vi "Draw Tree.vi"(8 "error in (no error)":errorcluster, 10 "Tree Data":T1(array[cluster]), 11 "Test Executive Builder View in":refnum<class "Test Executive Builder View.lvclass">) -> (0 "error out":errorcluster, 3 "Test Executive Builder View out":refnum<class "Test Executive Builder View.lvclass">)   [LabVIEW 2017, in "Test Executive Builder View.lvclass"]
uses:
  <vilib>/gpm_packages/@cs/Test-executive-builder/Source/Test Executive Builder View/Test Executive Builder View/Test Executive Builder View.lvclass
  <vilib>/gpm_packages/@cs/Test-executive-builder/Source/Test Executive Builder View/Test Executive Builder View/Test Executive Builder View.lvclass/Test Executive Builder View.ctl
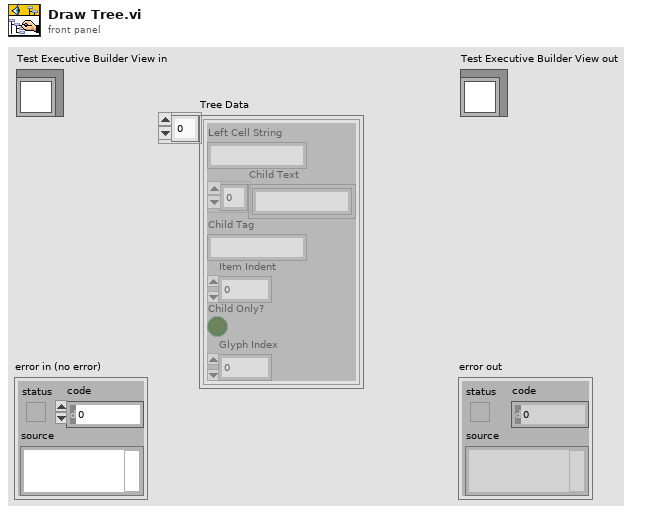
[diagram p1: front panel]
types:
  T1 = cluster{"Left Cell String":string, "Child Text":string[], "Child Tag":string, "Item Indent":i32, "Child Only?":bool, "Glyph Index":i32}[]
  T2 = typedef "LVNodeAndColumnTypeDef.ctl" = cluster{"Node":string, "Column":i32}
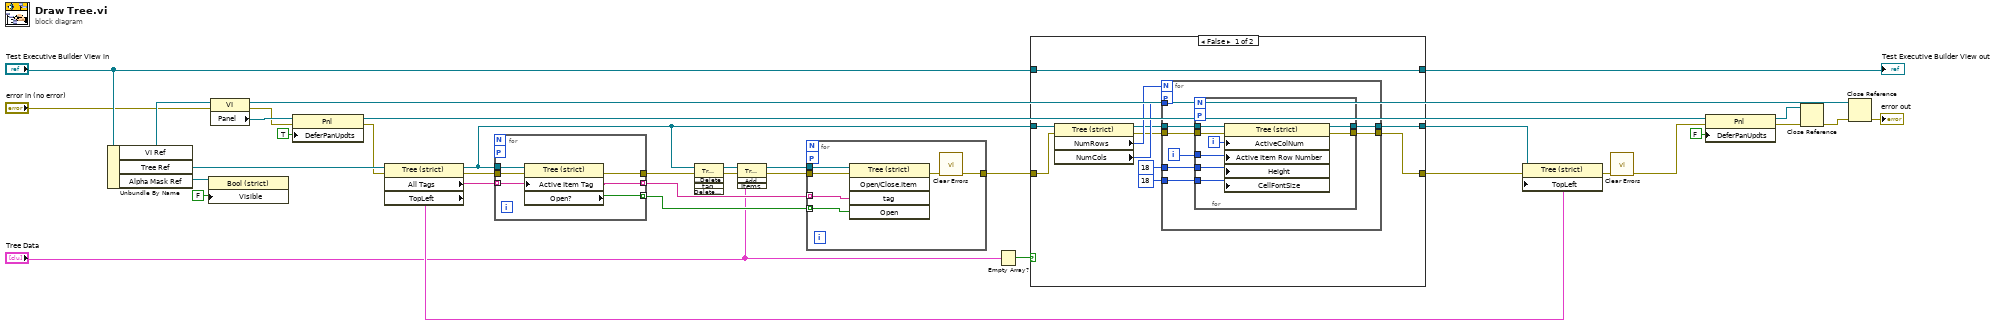
[diagram p0: block diagram]
diagram:
  n1 = Unbundle By Name("Test Executive Builder View in") -> ("VI Ref"=w36:refnum<vi>, "Tree Ref"=w32:refnum<vi>, "Alpha Mask Ref"=w11:refnum<vi>)
  n2 = property class="Bool (strict)"(reference=w11, "Visible"=FALSE) -> ()  [unwired: 1 in, 2 out]
  n3 = property class="VI"(reference=w36, error in="error in (no error)") -> (reference out=w15:refnum<vi>, error out=w33:errorcluster, "Panel"=w35:refnum<vi>)
  n4 = property class="Pnl"(reference=w35, error in=w33, "DeferPanUpdts"=TRUE ("Defer Panel Updates")) -> (reference out=w18:refnum<vi>, error out=w31:errorcluster)
  n5 = property class="Tree (strict)"(reference=w32, error in=w31) -> (reference out=w2:refnum<vi>, error out=w30:errorcluster, "All Tags"=w29:string[], "TopLeft"=w8:T2)
  n6 = for {
    tunnel: w29 -> [w37] mode=indexing
    tunnel: [w38] -> w23 mode=indexing
    tunnel: [w37] -> w22 mode=indexing
    tunnel: w30 -> [w40]
    tunnel: [w39] -> w28
    tunnel: w2 -> [w41]
    workers-P: _ -> [_]
    n7 = property class="Tree (strict)"(reference=w41, error in=w40, "Active Item Tag"=w37) -> (error out=w39:errorcluster, "Open?"=w38:bool)  [unwired: 1 out]
  }
  n8 = invoke class="Tree (strict)" method="Edit Tree Items.Delete"(reference=w2, error in=w28) -> (reference out=w27:refnum<vi>, error out=w26:errorcluster)  [unwired: 3 in, 3 out]
  n9 = invoke class="Tree (strict)" method="Edit Tree Items.Add Multiple Items to End"(reference=w27, error in=w26, "Items"="Tree Data") -> (reference out=w24:refnum<vi>, error out=w25:errorcluster)  [unwired: 1 in, 2 out]
  n10 = for {
    tunnel: w24 -> [w46]
    tunnel: w22 -> [w44] mode=indexing
    tunnel: w23 -> [w43] mode=indexing
    tunnel: w25 -> [w47]
    tunnel: [w42] -> w3
    workers-P: _ -> [_]
    n11 = invoke class="Tree (strict)" method="Open/Close.Item"(reference=w46, error in=w47, "tag"=w44, "Open"=w43) -> (error out=w45:errorcluster)  [unwired: 1 in, 4 out]
    n12 = call <vilib>:"Clear Errors.vi"("error in (no error)"=w45) -> ("error out"=w42:errorcluster)  [unwired: 5 in, 1 out]
  }
  n13 = Empty Array?(array="Tree Data") -> (empty?=w6:bool)
  n14 = case shown="False" w6 {
    tunnel: "Test Executive Builder View in" -> [w56 w77]
    tunnel: [w56 w77] -> w20
    tunnel: [w50 w76] -> w5
    tunnel: w3 -> [w57 w76]
    tunnel: w2 -> [w58 w75]
    tunnel: [w52 w75] -> w1
    frame False {
      n15 = property class="Tree (strict)"(reference=w58, error in=w57) -> (reference out=w53:refnum<vi>, error out=w51:errorcluster, "NumRows"=w55:u32, "NumCols"=w54:u32)
      n16 = for {
        N: w55 -> [_]
        tunnel: w54 -> [w66]
        workers-P: _ -> [_]
        tunnel: w53 -> [w65]
        tunnel: [w64] -> w52
        tunnel: w51 -> [w63]
        tunnel: [w62] -> w50
        tunnel: 18 ("Active Cell:Cell Size:Height") -> [w60]
        tunnel: u32 18 ("Active Cell:Cell Font:Size") -> [w59]
        i -> [w61]
        n17 = for {
          N: w66 -> [_]
          workers-P: _ -> [_]
          tunnel: w65 -> [w74]
          tunnel: [w73] -> w64
          tunnel: w63 -> [w72]
          tunnel: [w71] -> w62
          tunnel: w61 -> [w69]
          tunnel: w60 -> [w68]
          tunnel: w59 -> [w67]
          i -> [w70]
          n18 = property class="Tree (strict)"(reference=w74, error in=w72, "ActiveColNum"=w70, "Active Item Row Number"=w69, "Height"=w68, "CellFontSize"=w67) -> (reference out=w73:refnum<vi>, error out=w71:errorcluster)
        }
      }
    }
    frame True {
    }
  }
  "Test Executive Builder View out" <- w20
  n19 = property class="Tree (strict)"(reference=w1, error in=w5, "TopLeft"=w8) -> (error out=w9:errorcluster)  [unwired: 1 out]
  n20 = call <vilib>:"Clear Errors.vi"("error in (no error)"=w9) -> ("error out"=w4:errorcluster)  [unwired: 5 in, 1 out]
  n21 = property class="Pnl"(reference=w18, error in=w4, "DeferPanUpdts"=FALSE ("Defer Panel Updates")) -> (reference out=w17:refnum<vi>, error out=w16:errorcluster)
  n22 = Close Reference(reference=w17, error in (no error)=w16) -> (error out=w14:errorcluster)
  n23 = Close Reference(reference=w15, error in (no error)=w14) -> (error out=→"error out":errorcluster)
